vi "Python文件调用.vi"(10 "max_new_tokens":i32=100, 11 "text":string="面壁者") -> (0 "错误输出":errorcluster, 3 "out":string)   [LabVIEW 2024]
uses:
  <vilib>/Python/Open Anaconda Python Session.vi
panel:
  in  "Python version":string="3.9"
  in  "Env name":string="DL"
  in  "module path":path=path "D:/my_gpt8K_3/gpt_packet.py"
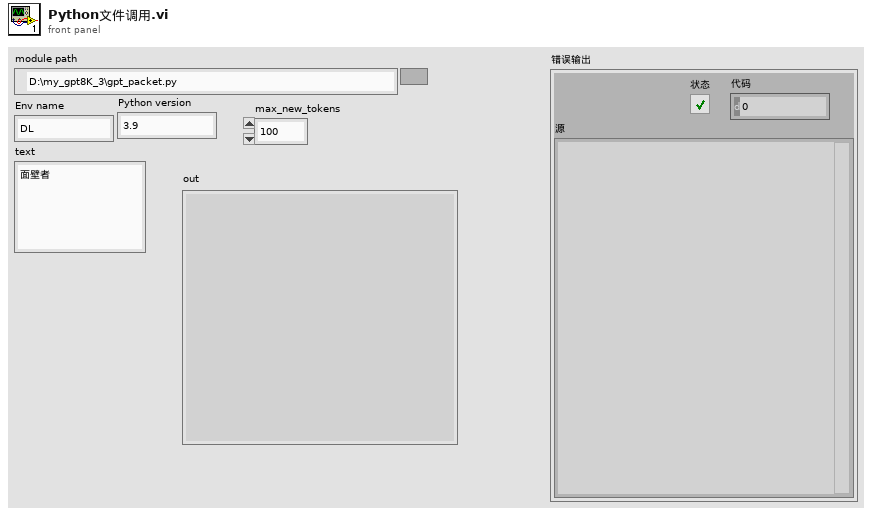
[diagram p1: front panel]
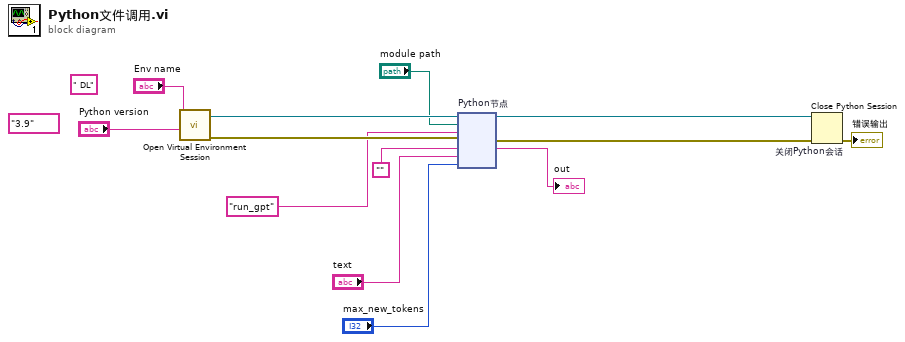
[diagram p0: block diagram]
diagram:
  (unwired) " DL" ("Env name")
  (unwired) "3.9" ("Python版本")
  n1 = call-poly <vilib>:"Open Virtual Environment Session.vi"("Python version"="Python version", "Env name"="Env name") -> ("error out"=w10:errorcluster, "session out"=w9:refnum<k35>)  [unwired: 8 in]
  n2 = node "Python节点"(w9, "module path", "run_gpt" ("函数名称"), w10, "", "text", "max_new_tokens") -> (w12:refnum<k35>, w13:errorcluster, →"out":string)  [unwired: 2 in, 2 out]
  n3 = Close Python Session "关闭Python会话"(session in=w12, error in=w13) -> (11:→"错误输出":errorcluster)
